vi "Pre Launch Init.vi"(11 "Nested in":refnum<class "Camera Worker.lvclass">) -> (0 "error out":errorcluster, 3 "Nested out":refnum<class "Camera Worker.lvclass">)   [LabVIEW 2024, in "Camera Worker.lvlib" / "Camera Worker.lvclass"]
doc: "(<B>Filename</B>: Actor Framework.lvlib:Actor.lvclass:Pre Launch Init.vi)\n\nDefines behavior that occurs after the Launch Nested Actor method is invoked but before the actor's Actor Core method begins running.\n\nBy default, this method does nothing. A descendant class may override it to define behavior."
uses:
  Camera Worker.lvclass
  Camera Worker.lvclass/Camera Worker.ctl
  Typedefs/Generic Image/Generic Image.lvclass
  <vilib>/ActorFramework/Actor/Actor.lvclass
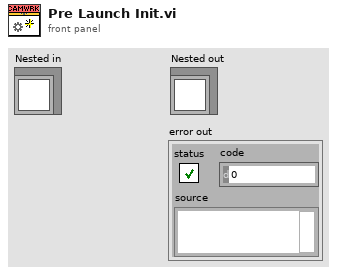
[diagram p1: front panel]
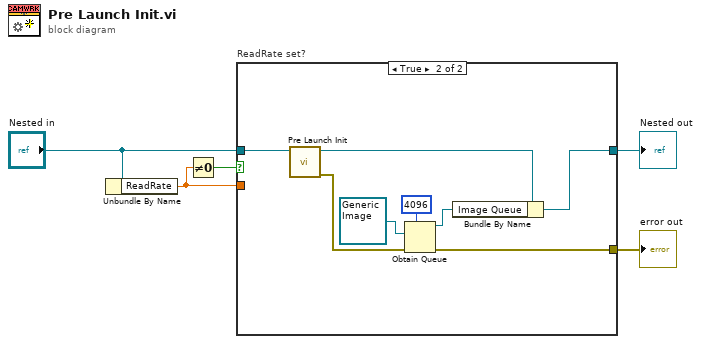
[diagram p0: block diagram]
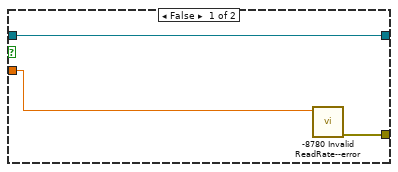
[diagram p2: hidden frame]
diagram:
  n1 = Unbundle By Name("Nested in") -> ("ReadRate"=w1:dbl)
  n2 = Not Equal To 0?(x=w1) -> (x != 0?=w2:bool)
  n3 = case "ReadRate set?" shown="True" w2 {
    tunnel: "Nested in" -> [w8 w14]
    tunnel: [w8 w16] -> w5
    tunnel: [w7 w15] -> w4
    tunnel: w1 -> [w6 _]
    frame False {
      n4 = call "-8780 Invalid ReadRate--error.vi"("Argument"=w6) -> ("error out"=w7:errorcluster)  [unwired: 10 in]
    }
    frame True {
      n5 = call-parent "Pre Launch Init.vi"("Actor in"=w14) -> ("error out"=w13:errorcluster, "Actor out"=w12:refnum<class "Camera Worker.lvclass">)  [unwired: 9 in]
      n6 = Obtain Queue(max queue size (-1, unlimited)=4096, element data type=refnum<class "Generic Image.lvclass"> refnum ("Generic Image.lvclass"), error in (no error)=w13) -> (queue out=w11:refnum<queue>, error out=w15:errorcluster)  [unwired: 2 in, 1 out]
      n7 = Bundle By Name(cluster=w12, "Image Queue"=w11) -> (w16:refnum<class "Camera Worker.lvclass">)
    }
  }
  "error out" <- w4
  "Nested out" <- w5
